vi "LogSpace (start-stop-n).vi"(0 "Start":dbl, 2 "Stop":dbl, 3 "N":i32) -> (6 "Array":dbl[](array[numeric]), 7 "error out":errorcluster)   [LabVIEW 2015]
uses:
  LinSpace (x0-dx-npts).vi
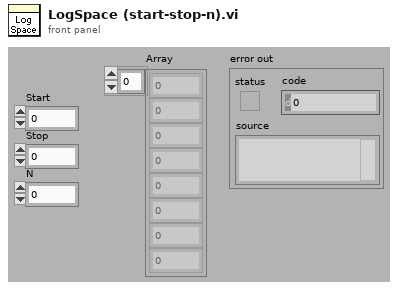
[diagram p1: front panel]
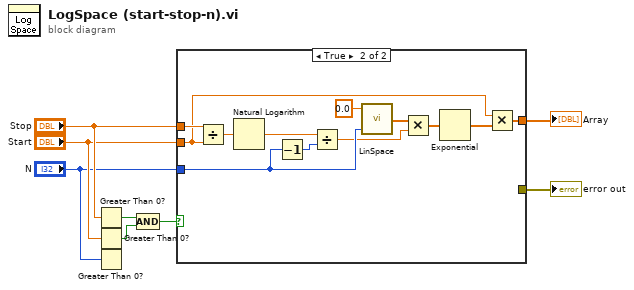
[diagram p0: block diagram]
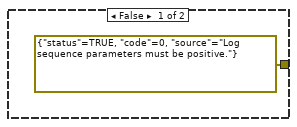
[diagram p2: hidden frame]
diagram:
  n1 = Greater Than 0?(x="Stop") -> (x > 0?=w4:bool)
  n2 = Greater Than 0?(x="Start") -> (x > 0?=w3:bool)
  n3 = Greater Than 0?(x="N") -> ()  [unwired: 1 out]
  n4 = Compound Arithmetic op=AND(w4, w3) -> (w2:bool)
  n5 = case shown="True" w2 {
    tunnel: [_ w19] -> w8
    tunnel: "Stop" -> [_ w18]
    tunnel: "Start" -> [_ w17]
    tunnel: "N" -> [_ w15]
    tunnel: [errorcluster {"status"=TRUE, "code"=0, "source"="Log sequence parameters must be positive."} ("error out") _] -> w1
    frame False {
    }
    frame True {
      n6 = Divide(x=w18, y=w17) -> (x/y=w11:dbl)
      n7 = Natural Logarithm(1:w11) -> (0:w10:dbl)
      n8 = Decrement(x=w15) -> (x-1=w16:i32)
      n9 = Divide(x=w10, y=w16) -> (x/y=w14:dbl)
      n10 = call-poly "LinSpace.vi"("npts"=w15, "x0"=0.0) -> ("Array"=w20:dbl[])  [unwired: 2 in, 1 out]
      n11 = Multiply(x=w20, y=w14) -> (x*y=w13:dbl[])
      n12 = Exponential(1:w13) -> (0:w12:dbl[])
      n13 = Multiply(x=w17, y=w12) -> (x*y=w19:dbl[])
    }
  }
  "Array" <- w8
  "error out" <- w1
